vi "RT_Example_Scripted.vi"() -> ()   [LabVIEW 2014]
uses:
  <vilib>/NI/cRIO Wfm/ChannelConfig.ctl
  <vilib>/FPGAPlugInAG/sbRIO-9651/niLvFpga_Open_sbRIO-9651.vi
  <vilib>/rvi/interface/common/dynamic/niFpgaDynamicAddResources.vi
  <vilib>/FPGAPlugInAG/Dynamic/niLvFpga_Reset_Dynamic.vi
  <vilib>/FPGAPlugInAG/Dynamic/niLvFpga_Run_Dynamic.vi
  <vilib>/NI/cRIO Wfm/AcqRead(Wfm).vi
  <vilib>/measure/matone.llb/Extract Single Tone Information 1 Chan.vi
  <vilib>/FPGAPlugInAG/Dynamic/niLvFpga_Close_Dynamic.vi
  <vilib>/rvi/interface/nirviOpenFPGA/nirviOpenFPGA.xnode
  FPGA Bitfiles/FPGAMainScripted.lvbitx
  <vilib>/rvi/interface/nirviMethod/nirviMethod.xnode
  <vilib>/rvi/interface/nirviCloseFPGA/nirviCloseFPGA.xnode
  <vilib>/NI/cRIO Wfm/cRIO Wfm.lvlib
  <vilib>/measure/NI_MAPro.lvlib
panel:
  out "Detected Frequencies":dbl[](array[numeric])
  in  "Samples per Channel":i32=100
  in  "Sampling Rate":u32=1000
  out "Waveform Graph":waveform(sgl)[](graph)
  in  "stop":bool
  # "Configuration Settings"
  # "Analysis"
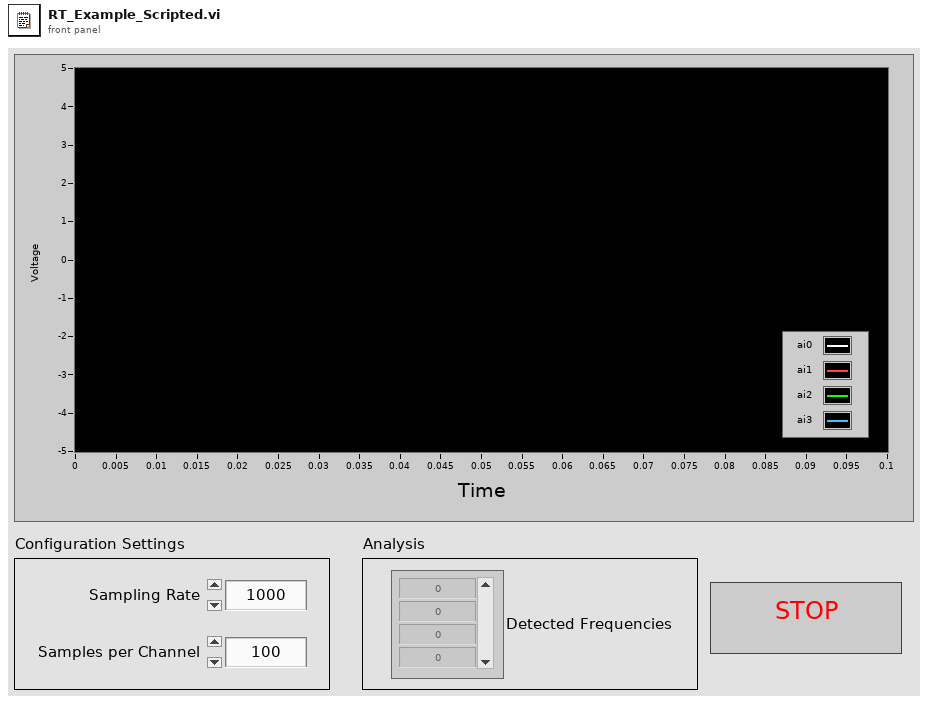
[diagram p1: front panel]
types:
  T1 = typedef "cRIO Wfm.lvlib/ChannelConfig.ctl" = cluster{"Channel Name":string, "Sensitivity mV_EU":dbl, "EU":string, "dB Ref EU":dbl}[]
  T2 = typedef "cRIO Wfm.lvlib/SamplingInfo.ctl" = cluster{"Number of Channels":i32, "Actual Samp Rate":dbl, "Chan Name Array":string[], "EU Chan Array":string[], "dB Ref Chan Array":dbl[]}
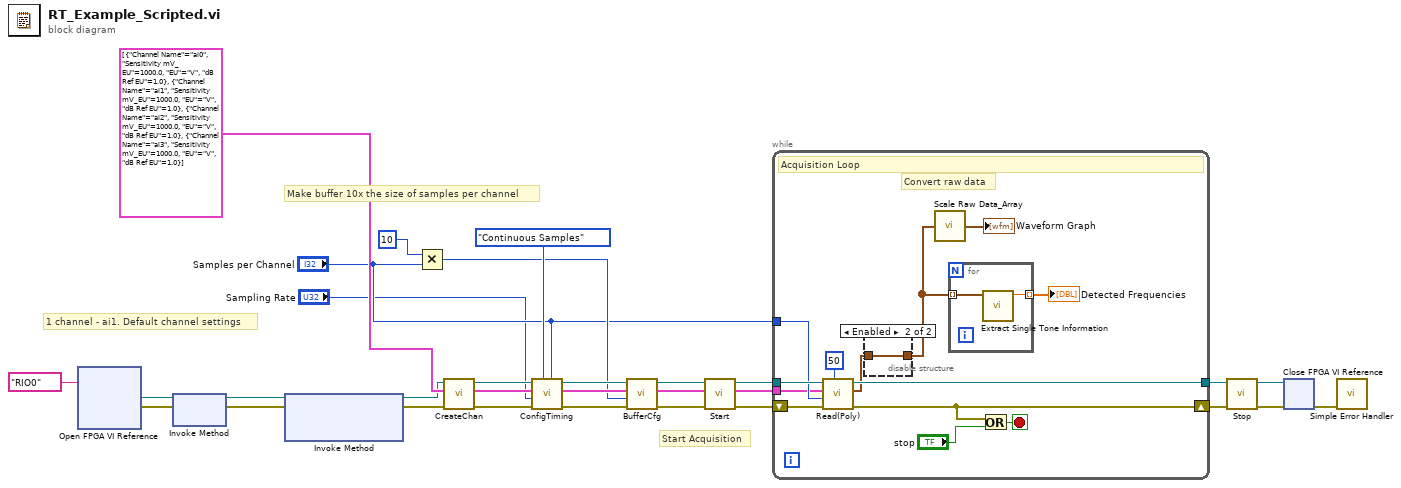
[diagram p0: block diagram]
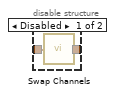
[diagram p2: hidden frame]
diagram:
  # "Start Acquisition"
  # "Make buffer 10x the size of samples per channel"
  # "1 channel - ai1. Default channel settings"
  n1 = xnode "Open FPGA VI Reference"("resource name"=tag "RIO0") -> ("FPGA VI Reference Out"=w30:refnum<k20>, "error out"=w29:errorcluster)  [unwired: 1 in]
  n2 = xnode "Invoke Method"("FPGA VI Reference In"=w30, "error in"=w29) -> ("FPGA VI Reference Out"=w3:refnum<k20>, "error out"=w2:errorcluster)
  n3 = xnode "Invoke Method"("FPGA VI Reference In"=w3, "error in"=w2) -> ("FPGA VI Reference Out"=w4:refnum<k20>, "error out"=w5:errorcluster)  [unwired: 1 in]
  n4 = Multiply(x=10 ("y"), y="Samples per Channel") -> (x*y=w13:i32)
  n5 = call <vilib>:"CreateChan.vi"("error in"=w5, "Channel Info"=T1 [{"Channel Name"="ai0", "Sensitivity mV_EU"=1000.0, "EU"="V", "dB Ref EU"=1.0}, {"Channel Name"="ai1", "Sensitivity mV_EU"=1000.0, "EU"="V", "dB Ref EU"=1.0}, {"Channel Name"="ai2", "Sensitivity mV_EU"=1000.0, "EU"="V", "dB Ref EU"=1.0}, {"Channel Name"="ai3", "Sensitivity mV_EU"=1000.0, "EU"="V", "dB Ref EU"=1.0}], "Dynamic FPGA Ref"=w4) -> ("error out"=w26:errorcluster, "Sampling Info"=w25:T2, "Dynamic FPGA Ref Out"=w28:refnum<k20>)  [unwired: 6 in]
  n6 = call <vilib>:"ConfigTiming.vi"("Samples per Channel"="Samples per Channel", "Sample Mode"=enum16{"Finite Samples", "Continuous Samples"}."Continuous Samples", "error in"=w26, "Sample Rate"="Sampling Rate", "Sampling Info In"=w25, "Dynamic FPGA Ref"=w28) -> ("error out"=w23:errorcluster, "Sampling Info Out"=w22:T2, "Dynamic FPGA Ref Out"=w24:refnum<k20>)  [unwired: 2 in, 1 out]
  n7 = call <vilib>:"BufferCfg.vi"("error in"=w23, "Buffer Size [Samps per Chan]"=w13, "Sampling Info In"=w22, "Dynamic FPGA Ref"=w24) -> ("error out"=w20:errorcluster, "Sampling Info Out"=w19:T2, "Dynamic FPGA Ref Out"=w21:refnum<k20>)  [unwired: 4 in, 1 out]
  n8 = call <vilib>:"Start.vi"("error in"=w20, "Sampling Info In"=w19, "Dynamic FPGA Ref"=w21) -> ("error out"=w7:errorcluster, "Sampling Info Out"=w10:T2, "Dynamic FPGA Ref Out"=w8:refnum<k20>)  [unwired: 6 in]
  n9 = while {
    tunnel: w8 -> [w43]
    shift-right: [w34] -> w17
    shift-left: w7 -> [w42]
    tunnel: [w41] -> w16
    tunnel: "Samples per Channel" -> [w40]
    tunnel: w10 -> [w39]
    stop <- w35 stop-if-true
    # "Convert raw data"
    # "Acquisition Loop"
    n10 = call-poly <vilib>:"Read(Poly).vi"("Poll Time (ms)"=u32 50, "error in"=w42, "Samps Read per Chan"=w40, "Sampling Info"=w39, "Dynamic FPGA Ref"=w43) -> ("error out"=w34:errorcluster, "Wfm Data"=w32:waveform(sgl)[], "Dynamic FPGA Ref Out"=w41:refnum<k20>)  [unwired: 3 in, 1 out]
    n11 = disable-structure shown="Enabled" {
      disable-tunnel: w32 -> [w45 w46]
      disable-tunnel: [w44 w46] -> w31
      frame Disabled {
        n12 = call "Swap Channels.vi"("Wfm Data"=w45) -> ("Wfm Data out"=w44:waveform(sgl)[])  [unwired: 14 in]
      }
      frame Enabled {
      }
    }
    n13 = call "Scale Raw Data_Array.vi"("Wfm Data"=w31) -> ("Wfm Data out"=→"Waveform Graph":waveform(sgl)[])  [unwired: 14 in]
    n14 = for {
      tunnel: w31 -> [w48] mode=indexing
      tunnel: [w47] -> w33 mode=indexing
      n15 = call-poly <vilib>:"Extract Single Tone Information.vi"("time signal in"=w48) -> ("detected frequency"=w47:dbl)  [unwired: 5 in, 5 out]
    }
    "Detected Frequencies" <- w33
    n16 = Or(x=w34, y="stop") -> (x .or. y?=w35:bool)
  }
  n17 = call <vilib>:"Stop.vi"("error in"=w17, "Dynamic FPGA Ref"=w16) -> ("error out"=w14:errorcluster, "Dynamic FPGA Ref Out"=w15:refnum<k20>)  [unwired: 8 in]
  n18 = xnode "Close FPGA VI Reference"("FPGA VI Reference In"=w15, "error in"=w14) -> ("error out"=w6:errorcluster)
  n19 = call <vilib>:"Simple Error Handler.vi"("error in (no error)"=w6) -> ()  [unwired: 4 in, 5 out]
